vi "GetTelemValue.vi"(7 "Not Found Value":string="-9999999", 8 "Telemetry In":cluster{"Name":string[], "Value":string[]}, 11 "Telemetry Name":string) -> (0 "Telemetry Out":cluster{"Name":string[], "Value":string[]}, 3 "Telemetry Value":string)   [LabVIEW 2015]
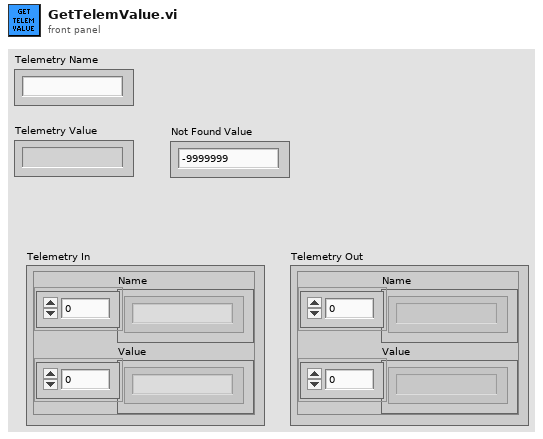
[diagram p1: front panel]
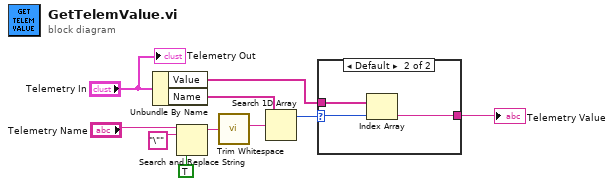
[diagram p0: block diagram]
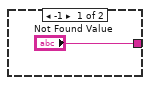
[diagram p2: hidden frame]
diagram:
  n1 = Unbundle By Name("Telemetry In") -> ("Value"=w2:string[], "Name"=w3:string[])
  n2 = Search and Replace String(replace all?=TRUE ("replace all? (F)"), input string="Telemetry Name", search string="\"") -> (result string=w7:string)  [unwired: 5 in, 3 out]
  n3 = call <vilib>:"Trim Whitespace.vi"("string"=w7) -> ("trimmed string"=w5:string)  [unwired: 1 in]
  n4 = Search 1D Array(1D array=w3, element=w5) -> (index of element=w4:i32)  [unwired: 1 in]
  n5 = case shown="Default" w4 {
    selector: w4 -> [_ w12]
    tunnel: w2 -> [_ w14]
    tunnel: ["Not Found Value" w13] -> w10
    frame -1 {
    }
    frame Default {
      n6 = Index Array(array=w14, index=w12) -> (element=w13:string)
    }
  }
  "Telemetry Value" <- w10
  "Telemetry Out" <- "Telemetry In"
